vi "Setting Database.GetPrivateEvents.vi"(8 "error in (no error)":errorcluster, 11 "Setting Database":refnum<class "Setting Database.lvclass">) -> (0 "error out":errorcluster, 2 "Private Events":T1, 3 "Setting Database out":refnum<class "Setting Database.lvclass">)   [LabVIEW 2019, in "Setting Database.lvclass"]
doc: "---------------------------------------------------------------\nJKI State Machine Objects™\nhttp://jki.net/state-machine-objects/\nCopyright (C) 2005-2015, JKI <info@jki.net>\nALL RIGHTS RESERVEDJKI State Machine Objects (SMO) 1.0.0.4\nJKI - JKI\nCopyright (c) 2015, JKI"
uses:
  Setting Database.lvclass
  Typedefs/PrivateEvents--Cluster.ctl
  Typedefs/PrivateEvents--Setting Database.SetActivePath.ctl
  Typedefs/PrivateEvents--Setting Database.UpdateActivePath.ctl
  Path Settings/Path Settings.lvclass
  Typedefs/PrivateEvents--Setting Database.Refresh.ctl
  Typedefs/PrivateEvents--Setting Database.CopyActivePathToAll.ctl
  Typedefs/PrivateEvents--Setting Database.SetActiveRectangle.ctl
  Typedefs/PrivateEvents--Setting Database.UpdateActiveRectangle.ctl
  Rectangle Settings/Rectangle Settings.lvclass
  Typedefs/PrivateEvents--Setting Database.CopyActiveRectangleToAll.ctl
  Typedefs/PrivateEvents--Setting Database.SetActiveFunnel.ctl
  Typedefs/PrivateEvents--Setting Database.UpdateActiveFunnel.ctl
  Funnel Settings/Funnel Settings.lvclass
  Typedefs/PrivateEvents--Setting Database.CopyActiveFunnelToAll.ctl
  Typedefs/PrivateEvents--Setting Database.SetDefaultPath.ctl
  Typedefs/PrivateEvents--Setting Database.SetDefaultRectangle.ctl
  Typedefs/PrivateEvents--Setting Database.SetDefaultFunnel.ctl
  Typedefs/PrivateEvents--Setting Database.SetDefaultDot.ctl
  Typedefs/PrivateEvents--Setting Database.SetActiveDot.ctl
  Typedefs/PrivateEvents--Setting Database.UpdateActiveDot.ctl
  Dot Settings/Dot Settings.lvclass
  Typedefs/PrivateEvents--Setting Database.CopyActiveDotToAll.ctl
  Typedefs/PrivateEvents--Setting Database.ChangeObjectEnable.ctl
  Setting Database.lvclass/Setting Database.ctl
panel:
  # "For instructions on how to use the JKI State Machine Objects, examples and video tutorials, visit:\nhttp://jki.net/state-machine-objects/\n\nJKI State Machine Objects™\nhttp://jki.net/state-machine-objects/\nCopyright (C) 2005-2015, JKI <info@jki.net>\nALL RIGHTS RESERVED"
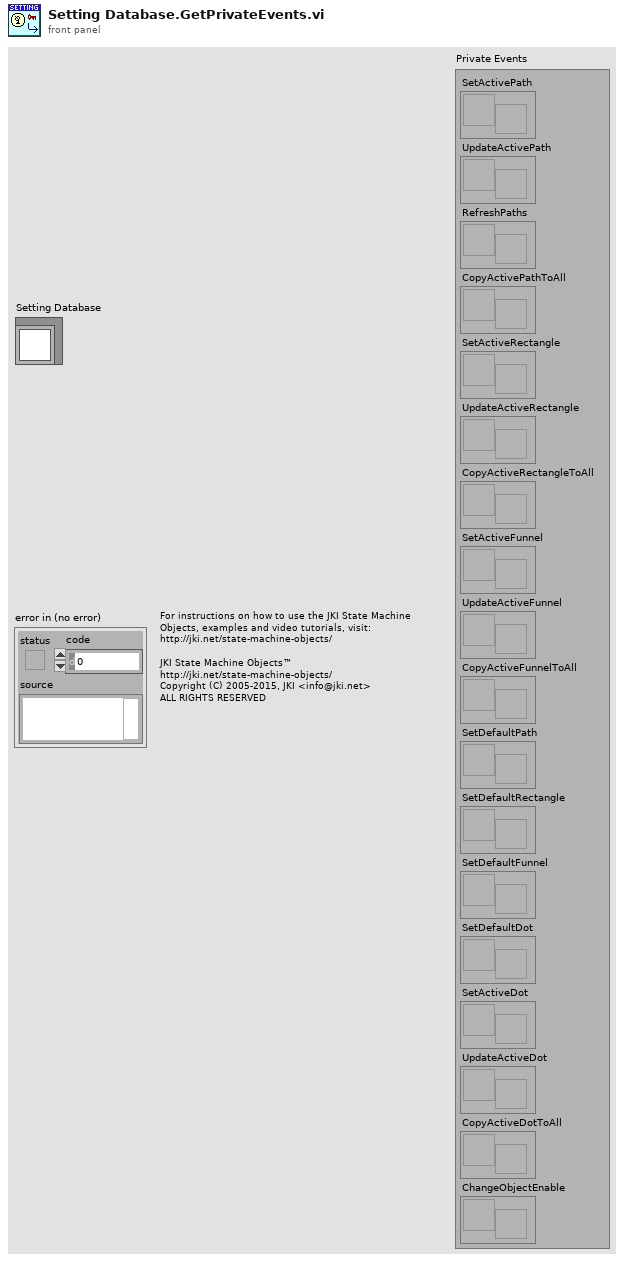
[diagram p1: front panel]
types:
  T1 = typedef "Setting Database.lvclass/PrivateEvents--Cluster.ctl" = cluster{"SetActivePath":refnum<user-event>, "UpdateActivePath":refnum<user-event>, "RefreshPaths":refnum<user-event>, "CopyActivePathToAll":refnum<user-event>, "SetActiveRectangle":refnum<user-event>, "UpdateActiveRectangle":refnum<user-event>, "CopyActiveRectangleToAll":refnum<user-event>, "SetActiveFunnel":refnum<user-event>, "UpdateActiveFunnel":refnum<user-event>, "CopyActiveFunnelToAll":refnum<user-event>, "SetDefaultPath":refnum<user-event>, "SetDefaultRectangle":refnum<user-event>, "SetDefaultFunnel":refnum<user-event>, "SetDefaultDot":refnum<user-event>, "SetActiveDot":refnum<user-event>, "UpdateActiveDot":refnum<user-event>, "CopyActiveDotToAll":refnum<user-event>, "ChangeObjectEnable":refnum<user-event>}
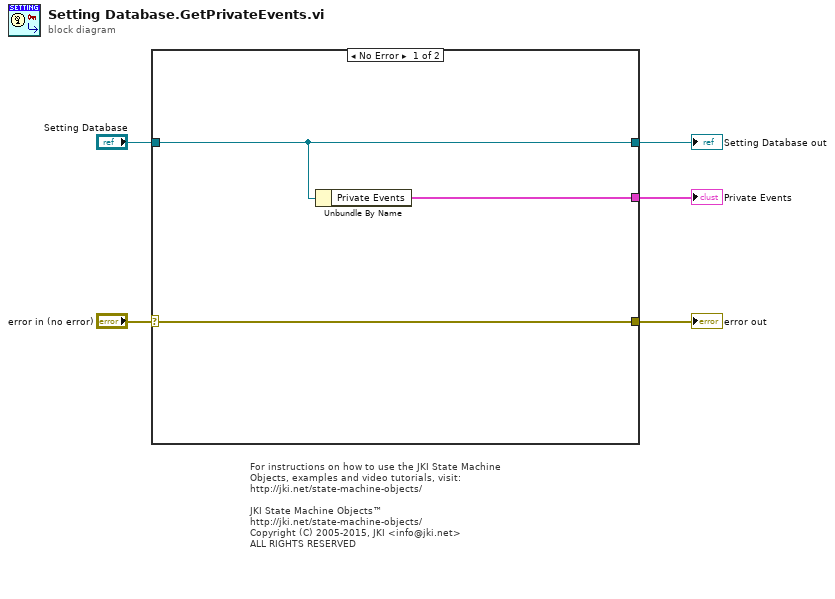
[diagram p0: block diagram]
diagram:
  # "For instructions on how to use the JKI State Machine Objects, examples and video tutorials, visit:\nhttp://jki.net/state-machine-objects/\n\nJKI State Machine Objects™\nhttp://jki.net/state-machine-objects/\nCopyright (C) 2005-2015, JKI <info@jki.net>\nALL RIGHTS RESERVED"
  n1 = case shown="No Error" "error in (no error)" {
    selector: "error in (no error)" -> [w7 w9]
    tunnel: "Setting Database" -> [w6 w10]
    tunnel: [w7 w9] -> w4
    tunnel: [w6 w10] -> w3
    tunnel: [w8 _] -> w1
    frame No Error {
      n2 = Unbundle By Name(w6) -> ("Private Events"=w8:T1)
    }
    frame Error {
    }
  }
  "error out" <- w4
  "Setting Database out" <- w3
  "Private Events" <- w1
